vi "Collate faulty sensor indices.vi"(8 "Error In":errorcluster, 11 "VISA resource name in":refnum<visa-resource-name>) -> (0 "Error out":errorcluster, 2 "Faulty sensor indices":i32[](array[numeric]), 3 "VISA resource name out":refnum<visa-resource-name>)   [LabVIEW 2015]
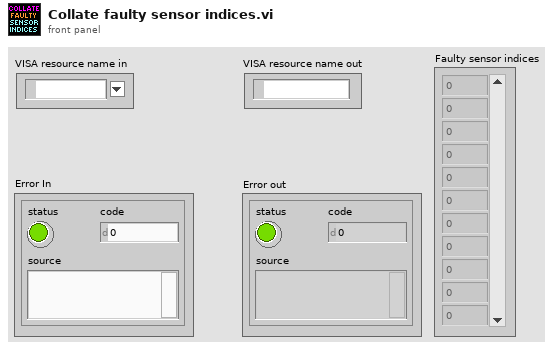
[diagram p1: front panel]
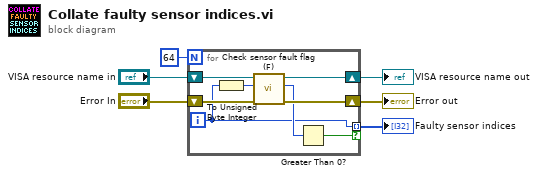
[diagram p0: block diagram]
diagram:
  n1 = for {
    N: 64 -> [_]
    shift-right: [w13] -> w5
    shift-left: "VISA resource name in" -> [w14]
    shift-right: [w11] -> w3
    shift-left: "Error In" -> [w12]
    tunnel: [w7] -> w1 mode=indexing if=w8
    i -> [w7]
    n2 = To Unsigned Byte Integer(number=w7) -> (unsigned 8bit integer=w10:u8)
    n3 = call "Check sensor fault flag (F).vi"("Error In"=w12, "Sensor index"=w10, "VISA resource name in"=w14) -> ("Error out"=w11:errorcluster, "Fault flag"=w9:u8, "VISA resource name out"=w13:refnum<visa-resource-name>)  [unwired: 5 in, 1 out]
    n4 = Greater Than 0?(x=w9) -> (x > 0?=w8:bool)
  }
  "VISA resource name out" <- w5
  "Error out" <- w3
  "Faulty sensor indices" <- w1
